vi "test.vi"() -> ()   [LabVIEW 2020, in "QuPMXdriver.lvlib"]
uses:
  QuPMXdriver.lvlib
panel:
  in  "Channel Guard Status":bool
  out "Delay (s) 2":dbl
  in  "Delay (s)":dbl=2.0
  out "Channel Enabled":bool
  in  "Channel Status":bool
  in  "Channel":i32=1 min=1 max=2 step=1
  in  "Slave":i32=1 min=1 max=6 step=1
  out "Enabled 2":bool
  out "Enabled":bool
  out "error out 2":errorcluster
  out "TRG External":bool
  out "TRG Polarity Positive":bool
  in  "Trigger Polarity Positive (T)":bool=TRUE
  in  "Trigger External (T)":bool=TRUE
  out "Internal Timer value (s)":dbl
  in  "Internal timer (2 s)":dbl=2.0 format="%#_10g"
  out "error out 3":errorcluster
  out "error out":errorcluster
  in  "Reset (True)":bool=TRUE
  in  "ID Query (True)":bool=TRUE
  in  "VISA resource name":refnum<visa-resource-name>
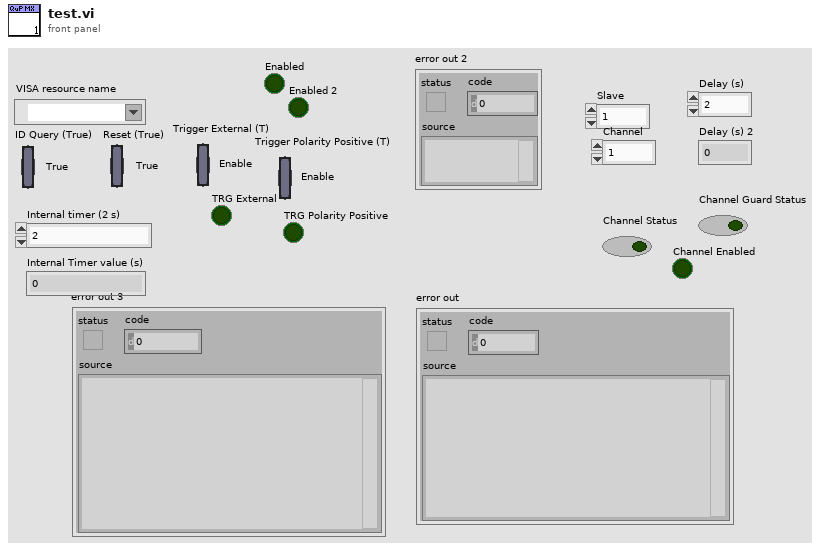
[diagram p1: front panel]
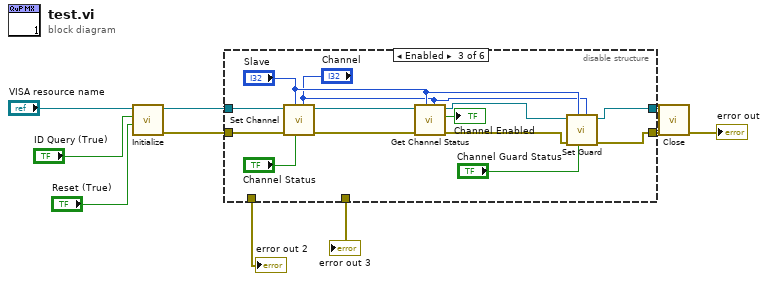
[diagram p0: block diagram]
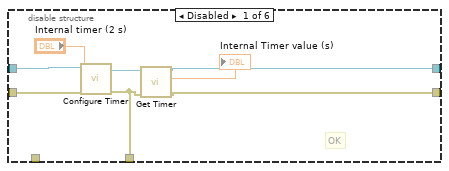
[diagram p2: hidden frame]
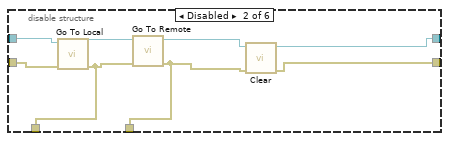
[diagram p3: hidden frame]
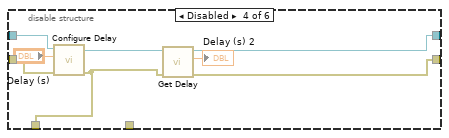
[diagram p4: hidden frame]
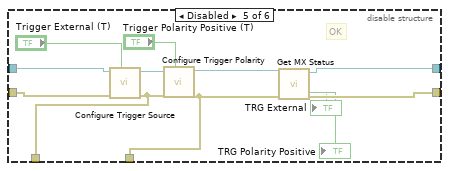
[diagram p5: hidden frame]
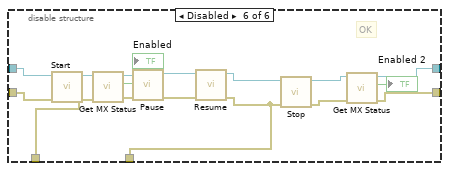
[diagram p6: hidden frame]
diagram:
  n1 = call "Initialize.vi"("Reset (True)"="Reset (True)", "ID Query (True)"="ID Query (True)", "VISA resource name"="VISA resource name") -> ("error out"=w6:errorcluster, "VISA resource name out"=w5:refnum<visa-resource-name>)  [unwired: 6 in, 1 out]
  n2 = disable-structure shown="Enabled" {
    disable-tunnel: w6 -> [w18 w26 w39 w47 w59 w75]
    disable-tunnel: w5 -> [w17 w25 w38 w42 w58 w74]
    disable-tunnel: [w15 w22 _ _ w49 w70] -> w4
    disable-tunnel: [w14 w21 w32 w45 w55 w63] -> w3
    disable-tunnel: [w13 w20 w31 w44 w54 w62] -> w2
    disable-tunnel: [_ w24 _ w46 w48 w69] -> w1
    frame Disabled {
      # "OK"
      n3 = call "Configure Timer.vi"("error in (no error)"=w18, "Internal timer (2 s)"="Internal timer (2 s)", "VISA resource name"=w17) -> ("error out"=w15:errorcluster, "VISA resource name out"=w11:refnum<visa-resource-name>)  [unwired: 7 in]
      n4 = call "Get Timer.vi"("error in (no error)"=w15, "VISA resource name"=w11) -> ("error out"=w14:errorcluster, "Internal Timer value (s)"=→"Internal Timer value (s)":dbl, "VISA resource name out"=w13:refnum<visa-resource-name>)  [unwired: 7 in]
    }
    frame Disabled {
      n5 = call "Go To Local.vi"("error in (no error)"=w26, "VISA resource name"=w25) -> ("error out"=w24:errorcluster, "VISA resource name out"=w23:refnum<visa-resource-name>)  [unwired: 8 in]
      n6 = call "Go To Remote.vi"("error in (no error)"=w24, "VISA resource name"=w23) -> ("error out"=w22:errorcluster, "VISA resource name out"=w19:refnum<visa-resource-name>)  [unwired: 8 in]
      n7 = call "Clear.vi"("error in (no error)"=w22, "VISA resource name"=w19) -> ("error out"=w21:errorcluster, "VISA resource name out"=w20:refnum<visa-resource-name>)  [unwired: 8 in]
    }
    frame Enabled {
      n8 = call "Set Channel.vi"("Channel"="Channel", "Channel Status"="Channel Status", "Slave"="Slave", "error in (no error)"=w39, "VISA resource name"=w38) -> ("error out"=w36:errorcluster, "VISA resource name out"=w35:refnum<visa-resource-name>)  [unwired: 5 in]
      n9 = call "Get Channel Status.vi"("Channel"="Channel", "Slave"="Slave", "error in (no error)"=w36, "VISA resource name"=w35) -> ("error out"=w33:errorcluster, "Channel Enabled"=→"Channel Enabled":bool, "VISA resource name out"=w30:refnum<visa-resource-name>)  [unwired: 5 in]
      n10 = call "Set Guard.vi"("Channel"="Channel", "Channel Guard Status"="Channel Guard Status", "Slave"="Slave", "error in (no error)"=w33, "VISA resource name"=w30) -> ("error out"=w32:errorcluster, "VISA resource name out"=w31:refnum<visa-resource-name>)  [unwired: 5 in]
    }
    frame Disabled {
      n11 = call "Configure Delay.vi"("error in (no error)"=w47, "Delay (s)"="Delay (s)", "VISA resource name"=w42) -> ("error out"=w46:errorcluster, "VISA resource name out"=w43:refnum<visa-resource-name>)  [unwired: 7 in]
      n12 = call "Get Delay.vi"("error in (no error)"=w46, "VISA resource name"=w43) -> ("error out"=w45:errorcluster, "Delay (s)"=→"Delay (s) 2":dbl, "VISA resource name out"=w44:refnum<visa-resource-name>)  [unwired: 7 in]
    }
    frame Disabled {
      # "OK"
      n13 = call "Configure Trigger Source.vi"("Trigger External (T)"="Trigger External (T)", "error in (no error)"=w59, "VISA resource name"=w58) -> ("error out"=w48:errorcluster, "VISA resource name out"=w57:refnum<visa-resource-name>)  [unwired: 7 in]
      n14 = call "Configure Trigger Polarity.vi"("Trigger Polarity Positive (T)"="Trigger Polarity Positive (T)", "error in (no error)"=w48, "VISA resource name"=w57) -> ("error out"=w49:errorcluster, "VISA resource name out"=w56:refnum<visa-resource-name>)  [unwired: 7 in]
      n15 = call "Get MX Status.vi"("error in (no error)"=w49, "VISA resource name"=w56) -> ("error out"=w55:errorcluster, "VISA resource name out"=w54:refnum<visa-resource-name>, "TRG Polarity Positive"=→"TRG Polarity Positive":bool, "TRG External"=→"TRG External":bool)  [unwired: 3 in, 3 out]
    }
    frame Disabled {
      # "OK"
      n16 = call "Start.vi"("error in (no error)"=w75, "VISA resource name"=w74) -> ("error out"=w69:errorcluster, "VISA resource name out"=w67:refnum<visa-resource-name>)  [unwired: 8 in]
      n17 = call "Get MX Status.vi"("error in (no error)"=w69, "VISA resource name"=w67) -> ("error out"=w68:errorcluster, "Enabled"=→"Enabled":bool, "VISA resource name out"=w66:refnum<visa-resource-name>)  [unwired: 3 in, 4 out]
      n18 = call "Pause.vi"("error in (no error)"=w68, "VISA resource name"=w66) -> ("error out"=w71:errorcluster, "VISA resource name out"=w73:refnum<visa-resource-name>)  [unwired: 8 in]
      n19 = call "Resume.vi"("error in (no error)"=w71, "VISA resource name"=w73) -> ("error out"=w70:errorcluster, "VISA resource name out"=w72:refnum<visa-resource-name>)  [unwired: 8 in]
      n20 = call "Stop.vi"("error in (no error)"=w70, "VISA resource name"=w72) -> ("error out"=w64:errorcluster, "VISA resource name out"=w61:refnum<visa-resource-name>)  [unwired: 8 in]
      n21 = call "Get MX Status.vi"("error in (no error)"=w64, "VISA resource name"=w61) -> ("error out"=w63:errorcluster, "Enabled"=→"Enabled 2":bool, "VISA resource name out"=w62:refnum<visa-resource-name>)  [unwired: 3 in, 4 out]
    }
  }
  "error out 3" <- w4
  "error out 2" <- w1
  n22 = call "Close.vi"("error in (no error)"=w3, "VISA resource name"=w2) -> ("error out"=→"error out":errorcluster)  [unwired: 9 in]
